vi "GE 5565PIORC.Close.vi"(8 "error in (no error)":errorcluster, 11 "GE 5565PIORC in":refnum<class "GE 5565PIORC.lvclass">) -> (0 "error out":errorcluster, 3 "VISA resource name out":refnum<visa-resource-name>)   [LabVIEW 2024, in "GE 5565PIORC.lvclass"]
doc: "Closes the current VISA session to the GE Reflective Memory card."
uses:
  GE 5565PIORC.lvclass
  GE 5565PIORC.lvclass/GE 5565PIORC.ctl
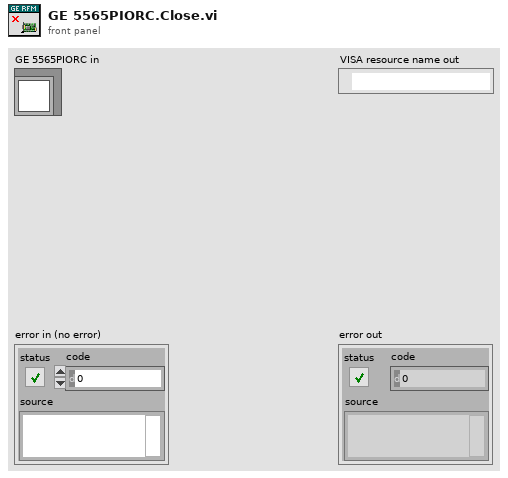
[diagram p1: front panel]
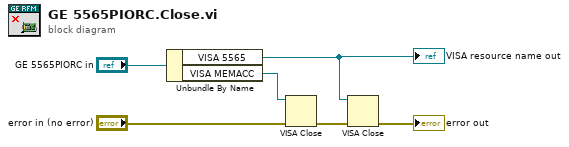
[diagram p0: block diagram]
diagram:
  n1 = Unbundle By Name("GE 5565PIORC in") -> ("VISA 5565"=w4:refnum<visa-resource-name>, "VISA MEMACC"=w6:refnum<visa-resource-name>)
  "VISA resource name out" <- w4
  n2 = VISA Close(VISA resource name=w6, error in (no error)="error in (no error)") -> (error out=w5:errorcluster)
  n3 = VISA Close(VISA resource name=w4, error in (no error)=w5) -> (error out=→"error out":errorcluster)
